vi "Open Connection.vi"(8 "error in (no error)":errorcluster, 11 "Client IP Address":string) -> (0 "error out":errorcluster, 3 "TCP Network Connection out":refnum<k5>)   [LabVIEW 2024, in "OptoMMP.lvlib"]
doc: "Opens a TCP/IP connection on port 2001 for communication via OptoMMP. \n\nThis is the first function to be used in any VI using the OptoMMP communication protocol.\n\nLast updated: 7/17/2025"
uses:
  <instrlib>/OptoMMP/OptoMMP.lvlib
panel:
  # "Copyright (c) 2025 California Institute of Technology (Caltech).\nU.S. Government sponsorship acknowledged.\n\nLicensed under the Apache License, Version 2.0 (the \"License\");\nyou may not use this file except in compliance with the License.\nYou may obtain a copy of the License at\n\n    http://www.apache.org/licenses/LICENSE-2.0\n\nUnless required by applicable law or agreed to in writing, software\ndistributed under the License is distributed on an \"AS IS\" BASIS,\nWITHOUT WARRANTIES OR CONDITIONS OF ANY KIND, either express or implied.\nSee the License for the specific language governing permissions and\nlimitations under the License."
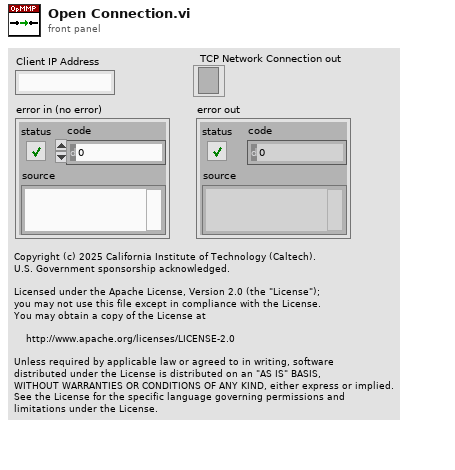
[diagram p1: front panel]
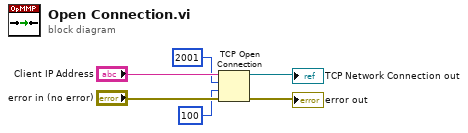
[diagram p0: block diagram]
diagram:
  n1 = TCP Open Connection(address="Client IP Address", remote port or service name=u16 2001, timeout ms (60000)=100, error in (no error)="error in (no error)") -> (connection ID=→"TCP Network Connection out":refnum<k5>, error out=→"error out":errorcluster)  [unwired: 1 in]
